vi "HEWH RLT PRAT.vi"() -> ()   [LabVIEW 2023] (continued)
        n1633 = call-poly "Enqueue Message.vi"("Priority Message? (F)"=TRUE, "error in (no error)"=w4189, "Message Data"="Temp (°F)", "Message"="Adjust_Temp_Intellifaucet_MW100", "Message Queue"=w4184) -> ("error out"=w4185:errorcluster)  [unwired: 5 in, 1 out]
      }
      frame "Adjust_Flow_Intellifaucet_MW100_UI" {
        n1634 = call-poly "Enqueue Message.vi"("Priority Message? (F)"=TRUE, "error in (no error)"=w4196, "Message Data"="Valve % Open", "Message"="Adjust_Flow_Intellifaucet_MW100", "Message Queue"=w4191) -> ("error out"=w4192:errorcluster)  [unwired: 5 in, 1 out]
      }
      frame "Adjust_Prop_Valve_MW100_UI" {
        n1635 = call-poly "Enqueue Message.vi"("Priority Message? (F)"=TRUE, "error in (no error)"=w4203, "Message Data"="Proportioning\nValve", "Message"="Adjust_Prop_Valve_MW100", "Message Queue"=w4198) -> ("error out"=w4199:errorcluster)  [unwired: 5 in, 1 out]
      }
      frame "DisplayValuesFromMW100" {
        # "Update Display - Convert the message data to a string to display in the Data Display indicator."
        n1636 = Variant To Data(error in=w4213, type=T79 {"TC1-Channel 021"=0.0, "TC2-Channel 022"=0.0, "TC3-Channel 023"=0.0, "TC4-Channel 024"=0.0, "TC5-Channel 025"=0.0, "TC6-Channel 026"=0.0, "TC7-Channel 017"=0.0, "TC8-Channel 028"=0.0, "TC9-Channel 029"=0.0, "TC10-Channel 030"=0.0, "TC Tree Average"=0.0, "TC DWN- Channel 027"=0.0, "RTDin-Channel 031"=0.0, "RTDout-Channel 032"=0.0, "RTDamb-Channel 033"=0.0, "PSI1-Channel 011"=0.0, "PSI2-Channel 012"=0.0, "PSI3-Channel 013"=0.0, "PSI4-Channel 014"=0.0, "UE State-Channel 015"=0.0, "LE State-Channel 016"=0.0, "Module 4 Relay Status Output"={"INTELLIFAUCET TEMP(T)/FLOW(F) (CH 041)"=FALSE, "INTELLIFAUCET READY (CH 042)"=FALSE, "INTELLIFAUCET START (CH 043)"=FALSE, "INTELLIFAUCET STOP (CH 044)"=FALSE, "MAIN POWER RELAY (CH 047)"=FALSE, "NOT USED (CH 045)"=FALSE, "NOT USED (CH 046)"=FALSE, "PURGE VALVE RELAY (CH 048)"=FALSE, "OUTLET VALVE RELAY (CH 049)"=FALSE, "INLET VALVE RELAY (CH 050)"=FALSE, "Intellifaucet (% Open)"=0.0, "Proportioning Valve (%Open)"=0.0, "Intellifaucet Temp Setpoint (F)"=0.0}} ("MW100 Data 2"), Variant=w4212) -> (data=w4209:T79, error out=w4207:errorcluster)
        n1637 = Bundle By Name(cluster=w4211, "MW100 Data"=w4209) -> (w4210:T67)
        n1638 = call-poly "Enqueue Message.vi"("error in (no error)"=w4207, "Message"="Process_Data", "Message Queue"=w4205) -> ("error out"=w4206:errorcluster)  [unwired: 7 in, 1 out]
        n1639 = Merge Errors(w4206) -> (w4214:errorcluster)
      }
      frame "---------- Tenney Control ----------" {
        # "Place holder, only for organization and readability"
        # "Initialize - All initialization work should take place in this message, since other loops can potentially enqueue messages that execute immediately after this one."
      }
      frame "Set_Tenney_IP_Name_UI" {
        n1640 = Variant To Data(error in=w4223, type="", Variant=w4221) -> (data=w4218:string, error out=w4222:errorcluster)
        n1641 = call-poly "Enqueue Message.vi"("Priority Message? (F)"=TRUE, "error in (no error)"=w4222, "Message Data"=w4218, "Message"="Set_Tenney_IP_Name", "Message Queue"=w4217) -> ("error out"=w4220:errorcluster)  [unwired: 5 in, 1 out]
      }
      frame "Tenney_Enable_Auto_Control_UI" {
        n1642 = Variant To Data(error in=w4231, type=TRUE, Variant=w4229) -> (data=w4228:bool, error out=w4230:errorcluster)
        n1643 = call-poly "Enqueue Message.vi"("Priority Message? (F)"=TRUE, "error in (no error)"=w4230, "Message Data"=w4228, "Message"="Tenney_Enable_Auto_Control", "Message Queue"=w4233) -> ("error out"=w4235:errorcluster)  [unwired: 5 in, 1 out]
        n1644 = Merge Errors(w4235) -> (w4236:errorcluster)
      }
      frame "PUT_Tenney_Temp_UI" {
        n1645 = call-poly "Enqueue Message.vi"("Priority Message? (F)"=TRUE, "error in (no error)"=w4243, "Message Data"="Setpoint Temperature (F)", "Message"="PUT_Tenney_Temp", "Message Queue"=w4240) -> ("error out"=w4242:errorcluster)  [unwired: 5 in, 1 out]
        n1646 = Merge Errors(w4242) -> (w4244:errorcluster)
      }
      frame "PUT_Tenney_Humidity_UI" {
        n1647 = call-poly "Enqueue Message.vi"("Priority Message? (F)"=TRUE, "error in (no error)"=w4251, "Message Data"="Setpoint Humidity (%)", "Message"="PUT_Tenney_Humidity", "Message Queue"=w4248) -> ("error out"=w4250:errorcluster)  [unwired: 5 in, 1 out]
        n1648 = Merge Errors(w4250) -> (w4252:errorcluster)
      }
      frame "PUT_Tenney_Frequency_UI" {
        n1649 = call-poly "Enqueue Message.vi"("Priority Message? (F)"=TRUE, "error in (no error)"=w4259, "Message Data"="Setpoint Frequency (Hz)", "Message"="PUT_Tenney_Frequency", "Message Queue"=w4256) -> ("error out"=w4258:errorcluster)  [unwired: 5 in, 1 out]
        n1650 = Merge Errors(w4258) -> (w4260:errorcluster)
      }
      frame "PUT_Chamber_Status_UI" {
        n1651 = Variant To Data(error in=w4266, type=Tenney_Chamber_Status."OFF" ("Chamber Status"), Variant=w4264) -> (data=w4262:T46, error out=w4265:errorcluster)
        n1652 = call-poly "Enqueue Message.vi"("Priority Message? (F)"=TRUE, "error in (no error)"=w4265, "Message Data"=w4262, "Message"="PUT_Chamber_Status", "Message Queue"=w4268) -> ("error out"=w4270:errorcluster)  [unwired: 5 in, 1 out]
        n1653 = Merge Errors(w4270) -> (w4271:errorcluster)
      }
      frame "Update_Temp_Limits_UI" {
        n1654 = call-poly "Enqueue Message.vi"("Priority Message? (F)"=TRUE, "error in (no error)"=w4274, "Message Data"="Temperature Limits", "Message"="Update_Temp_Limits", "Message Queue"=w4276) -> ("error out"=w4278:errorcluster)  [unwired: 5 in, 1 out]
        n1655 = Merge Errors(w4278) -> (w4279:errorcluster)
      }
      frame "DisplayValuesFromTenney" {
        # "Update Display - Convert the message data to a string to display in the Data Display indicator."
        n1656 = Variant To Data(error in=w4290, type=T69 {"Temperature Setpoint"=0.0, "Temperature Process Variable"=0.0, "Humidity Setpoint"=0.0, "Humidity Process Variable"=0.0, "Frequency Setpoint"=0.0, "Frequency Process Variable"=0.0, "Chamber Status (ON/OFF)"=""} ("Tenney Environmental Chamber Data"), Variant=w4289) -> (data=w4285:T69, error out=w4283:errorcluster)
        n1657 = Bundle By Name(cluster=w4287, "Tenney Data"=w4285) -> (w4286:T67)
        n1658 = call-poly "Enqueue Message.vi"("error in (no error)"=w4283, "Message"="Process_Data", "Message Queue"=w4281) -> ("error out"=w4282:errorcluster)  [unwired: 7 in, 1 out]
        n1659 = Merge Errors(w4282) -> (w4291:errorcluster)
      }
      frame "---------- GEA3 Control Station A ----------" {
        # "Place holder, only for organization and readability"
        # "Initialize - All initialization work should take place in this message, since other loops can potentially enqueue messages that execute immediately after this one."
      }
      frame "GEA3_StationA_Board_ID_UI" {
        n1660 = Variant To Data(error in=w4300, type=HEWH_GEA3_Board_ID."Board ID - 0" ("GEA3 Pink Bean Board Index (Station A)"), Variant=w4298) -> (data=w4296:T49, error out=w4299:errorcluster)
        n1661 = call-poly "Enqueue Message.vi"("Priority Message? (F)"=TRUE, "error in (no error)"=w4299, "Message Data"=w4296, "Message"="GEA3_StationA_Board_ID", "Message Queue"=w4294) -> ("error out"=w4297:errorcluster)  [unwired: 5 in, 1 out]
      }
      frame "Update_TankSP_Offset_StationA_UI" {
        n1662 = call-poly "Enqueue Message.vi"("Priority Message? (F)"=TRUE, "error in (no error)"=w4306, "Message Data"="TankSP Offset", "Message"="Update_TankSP_Offset_StationA", "Message Queue"=w4305) -> ("error out"=w4309:errorcluster)  [unwired: 5 in, 1 out]
        n1663 = Merge Errors(w4309) -> (w4310:errorcluster)
      }
      frame "Update_User_Setpoint_StationA_UI" {
        n1664 = call-poly "Enqueue Message.vi"("Priority Message? (F)"=TRUE, "error in (no error)"=w4314, "Message Data"="User Setpoint", "Message"="Update_User_Setpoint_StationA", "Message Queue"=w4313) -> ("error out"=w4317:errorcluster)  [unwired: 5 in, 1 out]
        n1665 = Merge Errors(w4317) -> (w4318:errorcluster)
      }
      frame "Update_Mode_StationA_UI" {
        n1666 = call-poly "Enqueue Message.vi"("Priority Message? (F)"=TRUE, "error in (no error)"=w4322, "Message Data"="Heating Mode.", "Message"="Update_Mode_StationA", "Message Queue"=w4321) -> ("error out"=w4325:errorcluster)  [unwired: 5 in, 1 out]
        n1667 = Merge Errors(w4325) -> (w4326:errorcluster)
      }
      frame "Update_Capacity_StationA_UI" {
        n1668 = call-poly "Enqueue Message.vi"("Priority Message? (F)"=TRUE, "error in (no error)"=w4330, "Message Data"="Capacity Setting", "Message"="Update_Capacity_StationA", "Message Queue"=w4329) -> ("error out"=w4333:errorcluster)  [unwired: 5 in, 1 out]
        n1669 = Merge Errors(w4333) -> (w4334:errorcluster)
      }
      frame "Update_Personality_StationA_UI" {
        n1670 = call-poly "Enqueue Message.vi"("Priority Message? (F)"=TRUE, "error in (no error)"=w4338, "Message Data"="Personality", "Message"="Update_Personality_StationA", "Message Queue"=w4337) -> ("error out"=w4341:errorcluster)  [unwired: 5 in, 1 out]
        n1671 = Merge Errors(w4341) -> (w4342:errorcluster)
      }
      frame "Reset_Control_Counter_StationA_UI" {
        n1672 = call-poly "Enqueue Message.vi"("Priority Message? (F)"=TRUE, "error in (no error)"=w4345, "Message"="Reset_Control_Counter_StationA", "Message Queue"=w4344) -> ("error out"=w4348:errorcluster)  [unwired: 6 in, 1 out]
        n1673 = Merge Errors(w4348) -> (w4349:errorcluster)
      }
      frame "Enable_EMV_List_StationA_UI" {
        n1674 = call-poly "Enqueue Message.vi"("Priority Message? (F)"=TRUE, "error in (no error)"=w4353, "Message Data"="Enable EMV ERD List", "Message"="Enable_EMV_List_StationA", "Message Queue"=w4352) -> ("error out"=w4356:errorcluster)  [unwired: 5 in, 1 out]
        n1675 = Merge Errors(w4356) -> (w4357:errorcluster)
      }
      frame "Enable_Inverter_List_StationA_UI" {
        n1676 = call-poly "Enqueue Message.vi"("Priority Message? (F)"=TRUE, "error in (no error)"=w4361, "Message Data"="Enable Inverter ERD List", "Message"="Enable_Inverter_List_StationA", "Message Queue"=w4360) -> ("error out"=w4364:errorcluster)  [unwired: 5 in, 1 out]
        n1677 = Merge Errors(w4364) -> (w4365:errorcluster)
      }
      frame "Enable_HeatPump_List_StationA_UI" {
        n1678 = call-poly "Enqueue Message.vi"("Priority Message? (F)"=TRUE, "error in (no error)"=w4369, "Message Data"="Enable Heat Pump ERD List", "Message"="Enable_HeatPump_List_StationA", "Message Queue"=w4368) -> ("error out"=w4372:errorcluster)  [unwired: 5 in, 1 out]
        n1679 = Merge Errors(w4372) -> (w4373:errorcluster)
      }
      frame "GEA3_Controls_UI" {
        n1680 = Variant To Data(error in=w4379, type=TRUE, Variant=w4375) -> (data=w4378:bool, error out=w4377:errorcluster)
        n1681 = case shown="True" w4378 {
          tunnel: w4377 -> [w4382 w4384]
          tunnel: [w4382 w4384] -> w4376
          frame False {
            w4383 = T87."Disabled and Grayed Out" ("Disabled")
            n1682 = property on="Update User Setpoint" class="Bool"("DisabledEnum"=w4383) -> ()  [unwired: 2 in, 2 out]
            n1683 = property on="Update Mode" class="Bool"("DisabledEnum"=w4383) -> ()  [unwired: 2 in, 2 out]
            n1684 = property on="Update TankSP Offset" class="Bool"("DisabledEnum"=w4383) -> ()  [unwired: 2 in, 2 out]
            n1685 = property on="Update Personality" class="Bool"("DisabledEnum"=w4383) -> ()  [unwired: 2 in, 2 out]
          }
          frame True {
            w4385 = T87."Enabled" ("Disabled")
            n1686 = property on="Update User Setpoint" class="Bool"("DisabledEnum"=w4385) -> ()  [unwired: 2 in, 2 out]
            n1687 = property on="Update Mode" class="Bool"("DisabledEnum"=w4385) -> ()  [unwired: 2 in, 2 out]
            n1688 = property on="Update TankSP Offset" class="Bool"("DisabledEnum"=w4385) -> ()  [unwired: 2 in, 2 out]
            n1689 = property on="Update Personality" class="Bool"("DisabledEnum"=w4385) -> ()  [unwired: 2 in, 2 out]
          }
        }
      }
      frame "DisplayValuesFromGEA_StationA" {
        # "Update Display - Convert the message data to a string to display in the Data Display indicator."
        n1690 = Variant To Data(error in=w4395, type=T76 {"ERD Data Input"={"Mixing Valve"={"T7 Temp (°F) - (0x40B9)"=0.0, "MixValveAbsoluteStepPosition - (0x400B)"=0, "Flow State - (0X4069)"=0, "T6 Temp (°F) - (0x406E)"=0.0}, "Standard ERDs"={"User UI Mode (0X4020)"="", "User Setpoint (0x4024)"=0, "Compressor (0x4068)"=FALSE, "Lower Element (0x4068)"=FALSE, "Upper Element (0x4068)"=FALSE, "Fan (0x4068)"=FALSE, "T1 Temp Lower Tank (°F) - (0x405F)"=0.0, "T2 Temp Upper Tank (°F) - (0x4060)"=0.0, "Line Voltage (0x4066)"=0, "MeasuredCurrent (0x4065)"=0.0, "Tank Setpoint (°F) - (0x4026)"=0, "Depletion - (0x40CB)"=0, "Personality - (0x0035)"=0}, "Heat Pump"={"EEV Position - (0X4067)"=0, "T3A TEMP EVAP IN (°F) - (0x4061)"=0.0, "T3B TEMP EVAP OUT (°F) -(0x4062)"=0.0, "T4 TEMP COMP DISCHARGE (°F) - (0x4063)"=0.0, "T5 TEMP AMBIENT (°F)- (0x4064)"=0.0, "Condensate Sensor - (0x40BC)"=0, "Fan (RPM) - (0xF073)"=0, "PWM (%) - (0xF056)"=0, "Compressor Speed (RPM) - (0xF093)"=0, "Compressor Target (RPM) - (0xF081)"=0, "Compressor Power (W) - (0xF092)"=0, "CPU Temperature (°F) - (0x40BA)"=0.0, "Board Temperature (°F) - (0x40BB)"=0.0}, "Inverter"={"Inverter IGBT Temp (°C) - (0xF280)"=0.0, "Inverter Chip Temp (°C) - (0xF284)"=0.0}}, "ERD Data"=[]} ("GEA3 Data"), Variant=w4394) -> (data=w4390:T76, error out=w4388:errorcluster)
        n1691 = Bundle By Name(cluster=w4392, "GEA Data - Station A"=w4390) -> (w4391:T67)
        n1692 = call-poly "Enqueue Message.vi"("error in (no error)"=w4388, "Message"="Process_Data", "Message Queue"=w4386) -> ("error out"=w4387:errorcluster)  [unwired: 7 in, 1 out]
        n1693 = Merge Errors(w4387) -> (w4396:errorcluster)
      }
      frame "---------- GEA3 Control Station B ----------" {
        # "Place holder, only for organization and readability"
        # "Initialize - All initialization work should take place in this message, since other loops can potentially enqueue messages that execute immediately after this one."
      }
      frame "GEA3_StationB_Board_ID_UI" {
        n1694 = Variant To Data(error in=w4405, type=HEWH_GEA3_Board_ID."Board ID - 0" ("GEA3 Pink Bean Board Index (Station A)"), Variant=w4403) -> (data=w4401:T49, error out=w4404:errorcluster)
        n1695 = call-poly "Enqueue Message.vi"("Priority Message? (F)"=TRUE, "error in (no error)"=w4404, "Message Data"=w4401, "Message"="GEA3_StationB_Board_ID", "Message Queue"=w4399) -> ("error out"=w4402:errorcluster)  [unwired: 5 in, 1 out]
      }
      frame "DisplayValuesFromGEA_StationB" {
        # "Update Display - Convert the message data to a string to display in the Data Display indicator."
        n1696 = Variant To Data(error in=w4418, type=T76 {"ERD Data Input"={"Mixing Valve"={"T7 Temp (°F) - (0x40B9)"=0.0, "MixValveAbsoluteStepPosition - (0x400B)"=0, "Flow State - (0X4069)"=0, "T6 Temp (°F) - (0x406E)"=0.0}, "Standard ERDs"={"User UI Mode (0X4020)"="", "User Setpoint (0x4024)"=0, "Compressor (0x4068)"=FALSE, "Lower Element (0x4068)"=FALSE, "Upper Element (0x4068)"=FALSE, "Fan (0x4068)"=FALSE, "T1 Temp Lower Tank (°F) - (0x405F)"=0.0, "T2 Temp Upper Tank (°F) - (0x4060)"=0.0, "Line Voltage (0x4066)"=0, "MeasuredCurrent (0x4065)"=0.0, "Tank Setpoint (°F) - (0x4026)"=0, "Depletion - (0x40CB)"=0, "Personality - (0x0035)"=0}, "Heat Pump"={"EEV Position - (0X4067)"=0, "T3A TEMP EVAP IN (°F) - (0x4061)"=0.0, "T3B TEMP EVAP OUT (°F) -(0x4062)"=0.0, "T4 TEMP COMP DISCHARGE (°F) - (0x4063)"=0.0, "T5 TEMP AMBIENT (°F)- (0x4064)"=0.0, "Condensate Sensor - (0x40BC)"=0, "Fan (RPM) - (0xF073)"=0, "PWM (%) - (0xF056)"=0, "Compressor Speed (RPM) - (0xF093)"=0, "Compressor Target (RPM) - (0xF081)"=0, "Compressor Power (W) - (0xF092)"=0, "CPU Temperature (°F) - (0x40BA)"=0.0, "Board Temperature (°F) - (0x40BB)"=0.0}, "Inverter"={"Inverter IGBT Temp (°C) - (0xF280)"=0.0, "Inverter Chip Temp (°C) - (0xF284)"=0.0}}, "ERD Data"=[]} ("GEA3 Data"), Variant=w4417) -> (data=w4413:T76, error out=w4411:errorcluster)
        n1697 = Bundle By Name(cluster=w4415, "GEA Data - Station B"=w4413) -> (w4414:T67)
        n1698 = call-poly "Enqueue Message.vi"("error in (no error)"=w4411, "Message"="Process_Data", "Message Queue"=w4409) -> ("error out"=w4410:errorcluster)  [unwired: 7 in, 1 out]
        n1699 = Merge Errors(w4410) -> (w4419:errorcluster)
      }
      frame "---------- GEA3 Control Station C ----------" {
        # "Place holder, only for organization and readability"
        # "Initialize - All initialization work should take place in this message, since other loops can potentially enqueue messages that execute immediately after this one."
      }
      frame "GEA3_StationC_Board_ID_UI" {
        n1700 = Variant To Data(error in=w4428, type=HEWH_GEA3_Board_ID."Board ID - 0" ("GEA3 Pink Bean Board Index (Station A)"), Variant=w4426) -> (data=w4424:T49, error out=w4427:errorcluster)
        n1701 = call-poly "Enqueue Message.vi"("Priority Message? (F)"=TRUE, "error in (no error)"=w4427, "Message Data"=w4424, "Message"="GEA3_StationC_Board_ID", "Message Queue"=w4422) -> ("error out"=w4425:errorcluster)  [unwired: 5 in, 1 out]
      }
      frame "DisplayValuesFromGEA_StationC" {
        # "Update Display - Convert the message data to a string to display in the Data Display indicator."
        n1702 = Variant To Data(error in=w4441, type=T76 {"ERD Data Input"={"Mixing Valve"={"T7 Temp (°F) - (0x40B9)"=0.0, "MixValveAbsoluteStepPosition - (0x400B)"=0, "Flow State - (0X4069)"=0, "T6 Temp (°F) - (0x406E)"=0.0}, "Standard ERDs"={"User UI Mode (0X4020)"="", "User Setpoint (0x4024)"=0, "Compressor (0x4068)"=FALSE, "Lower Element (0x4068)"=FALSE, "Upper Element (0x4068)"=FALSE, "Fan (0x4068)"=FALSE, "T1 Temp Lower Tank (°F) - (0x405F)"=0.0, "T2 Temp Upper Tank (°F) - (0x4060)"=0.0, "Line Voltage (0x4066)"=0, "MeasuredCurrent (0x4065)"=0.0, "Tank Setpoint (°F) - (0x4026)"=0, "Depletion - (0x40CB)"=0, "Personality - (0x0035)"=0}, "Heat Pump"={"EEV Position - (0X4067)"=0, "T3A TEMP EVAP IN (°F) - (0x4061)"=0.0, "T3B TEMP EVAP OUT (°F) -(0x4062)"=0.0, "T4 TEMP COMP DISCHARGE (°F) - (0x4063)"=0.0, "T5 TEMP AMBIENT (°F)- (0x4064)"=0.0, "Condensate Sensor - (0x40BC)"=0, "Fan (RPM) - (0xF073)"=0, "PWM (%) - (0xF056)"=0, "Compressor Speed (RPM) - (0xF093)"=0, "Compressor Target (RPM) - (0xF081)"=0, "Compressor Power (W) - (0xF092)"=0, "CPU Temperature (°F) - (0x40BA)"=0.0, "Board Temperature (°F) - (0x40BB)"=0.0}, "Inverter"={"Inverter IGBT Temp (°C) - (0xF280)"=0.0, "Inverter Chip Temp (°C) - (0xF284)"=0.0}}, "ERD Data"=[]} ("GEA3 Data"), Variant=w4440) -> (data=w4436:T76, error out=w4434:errorcluster)
        n1703 = Bundle By Name(cluster=w4438, "GEA Data - Station C"=w4436) -> (w4437:T67)
        n1704 = call-poly "Enqueue Message.vi"("error in (no error)"=w4434, "Message"="Process_Data", "Message Queue"=w4432) -> ("error out"=w4433:errorcluster)  [unwired: 7 in, 1 out]
        n1705 = Merge Errors(w4433) -> (w4442:errorcluster)
      }
      frame "---------- GEA3 Control Station D ----------" {
        # "Place holder, only for organization and readability"
        # "Initialize - All initialization work should take place in this message, since other loops can potentially enqueue messages that execute immediately after this one."
      }
      frame "GEA3_StationD_Board_ID_UI" {
        n1706 = Variant To Data(error in=w4451, type=HEWH_GEA3_Board_ID."Board ID - 0" ("GEA3 Pink Bean Board Index (Station A)"), Variant=w4449) -> (data=w4447:T49, error out=w4450:errorcluster)
        n1707 = call-poly "Enqueue Message.vi"("Priority Message? (F)"=TRUE, "error in (no error)"=w4450, "Message Data"=w4447, "Message"="GEA3_StationD_Board_ID", "Message Queue"=w4445) -> ("error out"=w4448:errorcluster)  [unwired: 5 in, 1 out]
      }
      frame "DisplayValuesFromGEA_StationD" {
        # "Update Display - Convert the message data to a string to display in the Data Display indicator."
        n1708 = Variant To Data(error in=w4464, type=T76 {"ERD Data Input"={"Mixing Valve"={"T7 Temp (°F) - (0x40B9)"=0.0, "MixValveAbsoluteStepPosition - (0x400B)"=0, "Flow State - (0X4069)"=0, "T6 Temp (°F) - (0x406E)"=0.0}, "Standard ERDs"={"User UI Mode (0X4020)"="", "User Setpoint (0x4024)"=0, "Compressor (0x4068)"=FALSE, "Lower Element (0x4068)"=FALSE, "Upper Element (0x4068)"=FALSE, "Fan (0x4068)"=FALSE, "T1 Temp Lower Tank (°F) - (0x405F)"=0.0, "T2 Temp Upper Tank (°F) - (0x4060)"=0.0, "Line Voltage (0x4066)"=0, "MeasuredCurrent (0x4065)"=0.0, "Tank Setpoint (°F) - (0x4026)"=0, "Depletion - (0x40CB)"=0, "Personality - (0x0035)"=0}, "Heat Pump"={"EEV Position - (0X4067)"=0, "T3A TEMP EVAP IN (°F) - (0x4061)"=0.0, "T3B TEMP EVAP OUT (°F) -(0x4062)"=0.0, "T4 TEMP COMP DISCHARGE (°F) - (0x4063)"=0.0, "T5 TEMP AMBIENT (°F)- (0x4064)"=0.0, "Condensate Sensor - (0x40BC)"=0, "Fan (RPM) - (0xF073)"=0, "PWM (%) - (0xF056)"=0, "Compressor Speed (RPM) - (0xF093)"=0, "Compressor Target (RPM) - (0xF081)"=0, "Compressor Power (W) - (0xF092)"=0, "CPU Temperature (°F) - (0x40BA)"=0.0, "Board Temperature (°F) - (0x40BB)"=0.0}, "Inverter"={"Inverter IGBT Temp (°C) - (0xF280)"=0.0, "Inverter Chip Temp (°C) - (0xF284)"=0.0}}, "ERD Data"=[]} ("GEA3 Data"), Variant=w4463) -> (data=w4459:T76, error out=w4457:errorcluster)
        n1709 = Bundle By Name(cluster=w4461, "GEA Data - Station D"=w4459) -> (w4460:T67)
        n1710 = call-poly "Enqueue Message.vi"("error in (no error)"=w4457, "Message"="Process_Data", "Message Queue"=w4455) -> ("error out"=w4456:errorcluster)  [unwired: 7 in, 1 out]
        n1711 = Merge Errors(w4456) -> (w4465:errorcluster)
      }
      frame "---------- Ultramat 23 Control ----------" {
        # "Place holder, only for organization and readability"
        # "Initialize - All initialization work should take place in this message, since other loops can potentially enqueue messages that execute immediately after this one."
      }
      frame "Set_Ultramat_VISA_Name_UI" {
        n1712 = Variant To Data(error in=w4474, type="", Variant=w4472) -> (data=w4468:string, error out=w4473:errorcluster)
        n1713 = call-poly "Enqueue Message.vi"("Priority Message? (F)"=TRUE, "error in (no error)"=w4473, "Message Data"=w4468, "Message"="Set_Ultramat_VISA_Name", "Message Queue"=w4470) -> ("error out"=w4471:errorcluster)  [unwired: 5 in, 1 out]
      }
      frame "DisplayValuesFromUltramat" {
        # "Update Display - Convert the message data to a string to display in the Data Display indicator."
        n1714 = Variant To Data(error in=w4487, type=string[][] [], Variant=w4486) -> (data=w4482:string[][], error out=w4480:errorcluster)
        n1715 = Bundle By Name(cluster=w4484, "Ultramat 23 Data"=w4482) -> (w4483:T67)
        n1716 = call-poly "Enqueue Message.vi"("error in (no error)"=w4480, "Message"="Process_Data", "Message Queue"=w4478) -> ("error out"=w4479:errorcluster)  [unwired: 7 in, 1 out]
        n1717 = Merge Errors(w4479) -> (w4488:errorcluster)
      }
      frame "---------- UI Control ----------" {
        # "Place holder, only for organization and readability"
        # "Initialize - All initialization work should take place in this message, since other loops can potentially enqueue messages that execute immediately after this one."
      }
      frame "Cancel_Draw_UI" {
        # "Initialize - All initialization work should take place in this message, since other loops can potentially enqueue messages that execute immediately after this one."
        n1718 = for {
          N: 10 -> [_]
          shift-right: [w4496] -> w4491
          shift-left: w4492 -> [w4497]
          n1719 = call "UTILITY Boolean Notifier.vi"("Status"=UTILITY_Notifier."Set", "error in (no error)"=w4497, "Set Status"=TRUE, "name (unnamed)"="Stop Custom Draw") -> ("error out"=w4496:errorcluster)  [unwired: 6 in, 1 out]
          n1720 = Wait Until Next ms Multiple(millisecond multiple=u32 10) -> ()  [unwired: 1 out]
        }
      }
      frame "DAQ_for_A_UI" {
        # "Initialize - All initialization work should take place in this message, since other loops can potentially enqueue messages that execute immediately after this one."
        n1721 = Variant To Data(error in=w4505, type=TRUE, Variant=w4501) -> (data=w4504:bool, error out=w4503:errorcluster)
        n1722 = case shown="True" w4504 {
          tunnel: w4503 -> [w4508 w4510]
          tunnel: [w4508 w4510] -> w4502
          frame False {
            w4509 = T87."Enabled" ("Disabled")
            n1723 = property on="DAQ for A" class="Bool (strict)"("DisabledEnum"=w4509) -> ()  [unwired: 2 in, 2 out]
            n1724 = property on="DAQ for B" class="Bool (strict)"("DisabledEnum"=w4509) -> ()  [unwired: 2 in, 2 out]
            n1725 = property on="DAQ for C" class="Bool (strict)"("DisabledEnum"=w4509) -> ()  [unwired: 2 in, 2 out]
            n1726 = property on="DAQ for D" class="Bool (strict)"("DisabledEnum"=w4509) -> ()  [unwired: 2 in, 2 out]
          }
          frame True {
            w4512 = T87."Disabled and Grayed Out" ("Disabled")
            n1727 = property on="DAQ for D" class="Bool (strict)"("DisabledEnum"=w4512) -> ()  [unwired: 2 in, 2 out]
            n1728 = property on="DAQ for B" class="Bool (strict)"("DisabledEnum"=w4512) -> ()  [unwired: 2 in, 2 out]
            n1729 = property on="DAQ for C" class="Bool (strict)"("DisabledEnum"=w4512) -> ()  [unwired: 2 in, 2 out]
            n1730 = property on="DAQ for A" class="Bool (strict)"("DisabledEnum"=T87."Enabled" ("Disabled")) -> ()  [unwired: 2 in, 2 out]
          }
        }
      }
      frame "DAQ_for_B_UI" {
        # "Initialize - All initialization work should take place in this message, since other loops can potentially enqueue messages that execute immediately after this one."
        n1731 = Variant To Data(error in=w4517, type=TRUE, Variant=w4513) -> (data=w4514:bool, error out=w4516:errorcluster)
        n1732 = case shown="True" w4514 {
          tunnel: w4516 -> [w4520 w4522]
          tunnel: [w4520 w4522] -> w4515
          frame False {
            w4521 = T87."Enabled" ("Disabled")
            n1733 = property on="DAQ for A" class="Bool (strict)"("DisabledEnum"=w4521) -> ()  [unwired: 2 in, 2 out]
            n1734 = property on="DAQ for B" class="Bool (strict)"("DisabledEnum"=w4521) -> ()  [unwired: 2 in, 2 out]
            n1735 = property on="DAQ for C" class="Bool (strict)"("DisabledEnum"=w4521) -> ()  [unwired: 2 in, 2 out]
            n1736 = property on="DAQ for D" class="Bool (strict)"("DisabledEnum"=w4521) -> ()  [unwired: 2 in, 2 out]
          }
          frame True {
            w4523 = T87."Disabled and Grayed Out" ("Disabled")
            n1737 = property on="DAQ for A" class="Bool (strict)"("DisabledEnum"=w4523) -> ()  [unwired: 2 in, 2 out]
            n1738 = property on="DAQ for C" class="Bool (strict)"("DisabledEnum"=w4523) -> ()  [unwired: 2 in, 2 out]
            n1739 = property on="DAQ for D" class="Bool (strict)"("DisabledEnum"=w4523) -> ()  [unwired: 2 in, 2 out]
            n1740 = property on="DAQ for B" class="Bool (strict)"("DisabledEnum"=T87."Enabled" ("Disabled")) -> ()  [unwired: 2 in, 2 out]
          }
        }
      }
      frame "DAQ_for_C_UI" {
        # "Initialize - All initialization work should take place in this message, since other loops can potentially enqueue messages that execute immediately after this one."
        n1741 = Variant To Data(error in=w4529, type=TRUE, Variant=w4525) -> (data=w4526:bool, error out=w4528:errorcluster)
        n1742 = case shown="False" w4526 {
          tunnel: w4528 -> [w4532 w4534]
          tunnel: [w4532 w4534] -> w4527
          frame False {
            w4533 = T87."Enabled" ("Disabled")
            n1743 = property on="DAQ for A" class="Bool (strict)"("DisabledEnum"=w4533) -> ()  [unwired: 2 in, 2 out]
            n1744 = property on="DAQ for D" class="Bool (strict)"("DisabledEnum"=w4533) -> ()  [unwired: 2 in, 2 out]
            n1745 = property on="DAQ for B" class="Bool (strict)"("DisabledEnum"=w4533) -> ()  [unwired: 2 in, 2 out]
            n1746 = property on="DAQ for C" class="Bool (strict)"("DisabledEnum"=w4533) -> ()  [unwired: 2 in, 2 out]
          }
          frame True {
            w4535 = T87."Disabled and Grayed Out" ("Disabled")
            n1747 = property on="DAQ for A" class="Bool (strict)"("DisabledEnum"=w4535) -> ()  [unwired: 2 in, 2 out]
            n1748 = property on="DAQ for B" class="Bool (strict)"("DisabledEnum"=w4535) -> ()  [unwired: 2 in, 2 out]
            n1749 = property on="DAQ for D" class="Bool (strict)"("DisabledEnum"=w4535) -> ()  [unwired: 2 in, 2 out]
            n1750 = property on="DAQ for C" class="Bool (strict)"("DisabledEnum"=T87."Enabled" ("Disabled")) -> ()  [unwired: 2 in, 2 out]
          }
        }
      }
      frame "DAQ_for_D_UI" {
        # "Initialize - All initialization work should take place in this message, since other loops can potentially enqueue messages that execute immediately after this one."
        n1751 = Variant To Data(error in=w4541, type=TRUE, Variant=w4537) -> (data=w4538:bool, error out=w4540:errorcluster)
        n1752 = case shown="False" w4538 {
          tunnel: w4540 -> [w4544 w4546]
          tunnel: [w4544 w4546] -> w4539
          frame False {
            w4545 = T87."Enabled" ("Disabled")
            n1753 = property on="DAQ for A" class="Bool (strict)"("DisabledEnum"=w4545) -> ()  [unwired: 2 in, 2 out]
            n1754 = property on="DAQ for B" class="Bool (strict)"("DisabledEnum"=w4545) -> ()  [unwired: 2 in, 2 out]
            n1755 = property on="DAQ for C" class="Bool (strict)"("DisabledEnum"=w4545) -> ()  [unwired: 2 in, 2 out]
            n1756 = property on="DAQ for D" class="Bool (strict)"("DisabledEnum"=w4545) -> ()  [unwired: 2 in, 2 out]
          }
          frame True {
            w4548 = T87."Disabled and Grayed Out" ("Disabled")
            n1757 = property on="DAQ for A" class="Bool (strict)"("DisabledEnum"=w4548) -> ()  [unwired: 2 in, 2 out]
            n1758 = property on="DAQ for B" class="Bool (strict)"("DisabledEnum"=w4548) -> ()  [unwired: 2 in, 2 out]
            n1759 = property on="DAQ for C" class="Bool (strict)"("DisabledEnum"=w4548) -> ()  [unwired: 2 in, 2 out]
            n1760 = property on="DAQ for D" class="Bool (strict)"("DisabledEnum"=T87."Enabled" ("Disabled")) -> ()  [unwired: 2 in, 2 out]
          }
        }
      }
      frame "Change_Gas_UI" {
        n1761 = call-poly "Enqueue Message.vi"("Priority Message? (F)"=TRUE, "error in (no error)"=w4559, "Message Data"="Gas Type", "Message"="Alicat_Change_Gas", "Message Queue"=w4555) -> ("error out"=w4553:errorcluster)  [unwired: 5 in, 1 out]
        n1762 = call-poly "Enqueue Message.vi"("Priority Message? (F)"=TRUE, "error in (no error)"=w4553, "Message Data"="Gas Type", "Message"="Ultramat_Select_Gas", "Message Queue"=w4551) -> ("error out"=w4552:errorcluster)  [unwired: 5 in, 1 out]
      }
      frame "Update_Graph_StationA_UI" {
        (unwired) 0 ("disabled index (col)")
        (unwired) 0 ("disabled index (col)")
        (unwired) 0 ("disabled index (col)")
        # "Initialize - All initialization work should take place in this message, since other loops can potentially enqueue messages that execute immediately after this one."
        n1763 = local read "Station A"() -> (w4562:string[][])
        n1764 = Transpose 2D Array(2D array=w4562) -> (transposed array=w4561:string[][])
        n1765 = Index Array(array=w4561) -> (element=w4565:string[])  [unwired: 2 in]
        n1766 = Index Array(array=w4561) -> (element=w4564:string[])  [unwired: 2 in]
        n1767 = Index Array(array=w4561) -> (element=w4563:string[])  [unwired: 2 in]
        n1768 = property on="X-Axis - Station A" class="CmbBox"("Strings[]"=w4565) -> ()  [unwired: 2 in, 2 out]
        n1769 = property on="Y-Axis1 - Station A" class="CmbBox"("Strings[]"=w4564) -> ()  [unwired: 2 in, 2 out]
        n1770 = property on="Y-Axis2 - Station A" class="CmbBox"("Strings[]"=w4563) -> ()  [unwired: 2 in, 2 out]
      }
      frame "Update_Graph_StationB_UI" {
        (unwired) 0 ("disabled index (col)")
        (unwired) 0 ("disabled index (col)")
        (unwired) 0 ("disabled index (col)")
        # "Initialize - All initialization work should take place in this message, since other loops can potentially enqueue messages that execute immediately after this one."
        n1771 = local read "Station B"() -> (w4568:string[][])
        n1772 = Transpose 2D Array(2D array=w4568) -> (transposed array=w4567:string[][])
        n1773 = Index Array(array=w4567) -> (element=w4571:string[])  [unwired: 2 in]
        n1774 = Index Array(array=w4567) -> (element=w4570:string[])  [unwired: 2 in]
        n1775 = Index Array(array=w4567) -> (element=w4569:string[])  [unwired: 2 in]
        n1776 = property on="X-Axis - Station B" class="CmbBox"("Strings[]"=w4571) -> ()  [unwired: 2 in, 2 out]
        n1777 = property on="Y-Axis1 - Station B" class="CmbBox"("Strings[]"=w4570) -> ()  [unwired: 2 in, 2 out]
        n1778 = property on="Y-Axis2 - Station B" class="CmbBox"("Strings[]"=w4569) -> ()  [unwired: 2 in, 2 out]
      }
      frame "Update_Graph_StationC_UI" {
        (unwired) 0 ("disabled index (col)")
        (unwired) 0 ("disabled index (col)")
        (unwired) 0 ("disabled index (col)")
        # "Initialize - All initialization work should take place in this message, since other loops can potentially enqueue messages that execute immediately after this one."
        n1779 = local read "Station C"() -> (w4575:string[][])
        n1780 = Transpose 2D Array(2D array=w4575) -> (transposed array=w4574:string[][])
        n1781 = Index Array(array=w4574) -> (element=w4578:string[])  [unwired: 2 in]
        n1782 = Index Array(array=w4574) -> (element=w4577:string[])  [unwired: 2 in]
        n1783 = Index Array(array=w4574) -> (element=w4576:string[])  [unwired: 2 in]
        n1784 = property on="X-Axis - Station C" class="CmbBox"("Strings[]"=w4578) -> ()  [unwired: 2 in, 2 out]
        n1785 = property on="Y-Axis1 - Station C" class="CmbBox"("Strings[]"=w4577) -> ()  [unwired: 2 in, 2 out]
        n1786 = property on="Y-Axis2 - Station C" class="CmbBox"("Strings[]"=w4576) -> ()  [unwired: 2 in, 2 out]
      }
      frame "Update_Graph_StationD_UI" {
        (unwired) 0 ("disabled index (col)")
        (unwired) 0 ("disabled index (col)")
        (unwired) 0 ("disabled index (col)")
        # "Initialize - All initialization work should take place in this message, since other loops can potentially enqueue messages that execute immediately after this one."
        n1787 = local read "Station D"() -> (w4581:string[][])
        n1788 = Transpose 2D Array(2D array=w4581) -> (transposed array=w4582:string[][])
        n1789 = Index Array(array=w4582) -> (element=w4585:string[])  [unwired: 2 in]
        n1790 = Index Array(array=w4582) -> (element=w4584:string[])  [unwired: 2 in]
        n1791 = Index Array(array=w4582) -> (element=w4583:string[])  [unwired: 2 in]
        n1792 = property on="X-Axis - Station D" class="CmbBox"("Strings[]"=w4585) -> ()  [unwired: 2 in, 2 out]
        n1793 = property on="Y-Axis1 - Station D" class="CmbBox"("Strings[]"=w4584) -> ()  [unwired: 2 in, 2 out]
        n1794 = property on="Y-Axis2 - Station D" class="CmbBox"("Strings[]"=w4583) -> ()  [unwired: 2 in, 2 out]
      }
      frame "---------- Alicat Gas Meter ----------" {
        # "Place holder, only for organization and readability"
        # "Initialize - All initialization work should take place in this message, since other loops can potentially enqueue messages that execute immediately after this one."
      }
      frame "Set_Alicat_VISA_Name_UI" {
        n1795 = Variant To Data(error in=w4596, type="", Variant=w4594) -> (data=w4591:string, error out=w4595:errorcluster)
        n1796 = call-poly "Enqueue Message.vi"("Priority Message? (F)"=TRUE, "error in (no error)"=w4595, "Message Data"=w4591, "Message"="Set_Alicat_VISA_Name", "Message Queue"=w4590) -> ("error out"=w4593:errorcluster)  [unwired: 5 in, 1 out]
      }
      frame "Alicat_Tare_Flow_UI" {
        n1797 = call-poly "Enqueue Message.vi"("Priority Message? (F)"=TRUE, "error in (no error)"=w4605, "Message"="Alicat_Tare_Flow", "Message Queue"=w4601) -> ("error out"=w4600:errorcluster)  [unwired: 6 in, 1 out]
      }
      frame "DisplayValuesFromAlicat" {
        # "Update Display - Convert the message data to a string to display in the Data Display indicator."
        n1798 = Variant To Data(error in=w4615, type=T71 {"Data Cluster"={"Absolute Pressure"=0.0, "Gauge/Diff. Pressure"=0.0, "Barometric Pressure"=0.0, "Temperature"=0.0, "Volumetric Flow"=0.0, "Mass Flow"=0.0, "Setpoint"=0.0, "Valve Drive"=0.0, "Totalizer"=0.0, "[hr]"=0.0, "[min]"=0.0, "[sec]"=0.0, "Totalizer Average Flow"=0.0, "Totalizer Peak Flow"=0.0, "Gas selected"=""}, "Units of Measure Input"={"Abs. Pressure"="", "Gauge/Diff. Press."="", "Barometric Press."="", "Temperature"="", "Volume"="", "Mass"="", "Setpoint"="", "Valve Drive"="", "Totalizer"="", "Tot. Timer"="", "Tot. Avg. Flow"="", "Tot. Peak Flow"=""}, "Header Array"=[]} ("Gas Data"), Variant=w4614) -> (data=w4610:T71, error out=w4608:errorcluster)
        n1799 = Bundle By Name(cluster=w4612, "Alicat Data"=w4610) -> (w4611:T67)
        n1800 = call-poly "Enqueue Message.vi"("error in (no error)"=w4608, "Message"="Process_Data", "Message Queue"=w4606) -> ("error out"=w4607:errorcluster)  [unwired: 7 in, 1 out]
        n1801 = Merge Errors(w4607) -> (w4616:errorcluster)
      }
      frame "---------- Wet Gas Meter ----------" {
        # "Place holder, only for organization and readability"
        # "Initialize - All initialization work should take place in this message, since other loops can potentially enqueue messages that execute immediately after this one."
      }
      frame "Set_Ritter_VISA_Name_UI" {
        n1802 = Variant To Data(error in=w4625, type="", Variant=w4623) -> (data=w4620:string, error out=w4624:errorcluster)
        n1803 = call-poly "Enqueue Message.vi"("Priority Message? (F)"=TRUE, "error in (no error)"=w4624, "Message Data"=w4620, "Message"="Set_Ritter_VISA_Name", "Message Queue"=w4619) -> ("error out"=w4622:errorcluster)  [unwired: 5 in, 1 out]
      }
      frame "Reset_Gas_Totalizer_UI" {
        w4633 = TRUE ("Priority Message? (F)")
        n1804 = call-poly "Enqueue Message.vi"("Priority Message? (F)"=w4633, "error in (no error)"=w4637, "Message"="Alicat_Tare_Totalizer", "Message Queue"=w4630) -> ("error out"=w4635:errorcluster)  [unwired: 6 in, 1 out]
        n1805 = call-poly "Enqueue Message.vi"("Priority Message? (F)"=w4633, "error in (no error)"=w4635, "Message"="Ritter_Tare_Totalizer", "Message Queue"=w4629) -> ("error out"=w4634:errorcluster)  [unwired: 6 in, 1 out]
      }
      frame "DisplayValuesFromRitter" {
        w4645 = T1 {"Gas Flow Rate (L/hr)-Uncorrected"=0.0, "Totalized Flow (L)--Uncorrected"=0.0, "Gas Flow Rate (cuft/hr)-Uncorrected"=0.0, "Totalized Flow (cuft)-Uncorrected"=0.0, "Gas Temperature (F)"=0.0, "Gas Pressure (in WC)"=0.0, "Heise Barometric Pressure (inHG)"=0.0, "STP Correction Factor"=0.0, "Temp Correction Factor"=0.0, "Pressure Correction Factor"=0.0, "Water Vapor Pressure"=0.0, "Gas Flow Rate (cuft/hr)-Corrected"=0.0, "Totalized Flow (cuft)-Corrected"=0.0, "Gas BTU"=0.0, "Gas BTU/hr"=0.0, "Gas Flow Rate (cuft/hr)-Uncorrected-Raw"=0.0}  # Gas Measurment Data - Ritter
        # "Update Display - Convert the message data to a string to display in the Data Display indicator."
        n1806 = Variant To Data(error in=w4647, type=w4645, Variant=w4646) -> (data=w4642:T1, error out=w4640:errorcluster)
        n1807 = Bundle By Name(cluster=w4644, "Ritter Data"=w4642) -> (w4643:T67)
        n1808 = call-poly "Enqueue Message.vi"("error in (no error)"=w4640, "Message"="Process_Data", "Message Queue"=w4638) -> ("error out"=w4639:errorcluster)  [unwired: 7 in, 1 out]
        n1809 = Merge Errors(w4639) -> (w4648:errorcluster)
      }
      frame "---------- Laurel Water Meter Control ----------" {
        # "Place holder, only for organization and readability"
        # "Initialize - All initialization work should take place in this message, since other loops can potentially enqueue messages that execute immediately after this one."
      }
      frame "Set_Laurel_IP_Name_UI" {
        n1810 = Variant To Data(error in=w4657, type="", Variant=w4655) -> (data=w4652:string, error out=w4656:errorcluster)
        n1811 = call-poly "Enqueue Message.vi"("Priority Message? (F)"=TRUE, "error in (no error)"=w4656, "Message Data"=w4652, "Message"="Set_Laurel_IP_Name", "Message Queue"=w4651) -> ("error out"=w4654:errorcluster)  [unwired: 5 in, 1 out]
      }
      frame "DisplayValuesFromLaurel" {
        # "Update Display - Convert the message data to a string to display in the Data Display indicator."
        n1812 = Variant To Data(error in=w4670, type=T73 {"Flow Rate (GPM)"=0.0, "Totalized Flow (Gallons)"=0.0} ("Laurel Meter Data"), Variant=w4669) -> (data=w4665:T73, error out=w4663:errorcluster)
        n1813 = Bundle By Name(cluster=w4667, "Laurel Meter Data"=w4665) -> (w4666:T67)
        n1814 = call-poly "Enqueue Message.vi"("error in (no error)"=w4663, "Message"="Process_Data", "Message Queue"=w4661) -> ("error out"=w4662:errorcluster)  [unwired: 7 in, 1 out]
        n1815 = Merge Errors(w4662) -> (w4671:errorcluster)
      }
      frame "---------- Emerson Water Meter Control ----------" {
        # "Place holder, only for organization and readability"
        # "Initialize - All initialization work should take place in this message, since other loops can potentially enqueue messages that execute immediately after this one."
      }
      frame "Set_Emerson_IP_Name_UI" {
        n1816 = Variant To Data(error in=w4680, type="", Variant=w4678) -> (data=w4675:string, error out=w4679:errorcluster)
        n1817 = call-poly "Enqueue Message.vi"("Priority Message? (F)"=TRUE, "error in (no error)"=w4679, "Message Data"=w4675, "Message"="Set_Emerson_IP_Name", "Message Queue"=w4674) -> ("error out"=w4677:errorcluster)  [unwired: 5 in, 1 out]
      }
      frame "Reset_Inventory_Emerson_UI" {
        n1818 = call-poly "Enqueue Message.vi"("Priority Message? (F)"=TRUE, "error in (no error)"=w4689, "Message"="Reset_Inventory_Emerson", "Message Queue"=w4684) -> ("error out"=w4685:errorcluster)  [unwired: 6 in, 1 out]
      }
      frame "Reset_Totalizer_UI" {
        n1819 = call-poly "Enqueue Message.vi"("Priority Message? (F)"=TRUE, "error in (no error)"=w4699, "Message"="Reset_Totalizer_Emerson", "Message Queue"=w4695) -> ("error out"=w4692:errorcluster)  [unwired: 6 in, 1 out]
        n1820 = call-poly "Enqueue Message.vi"("Priority Message? (F)"=TRUE, "error in (no error)"=w4692, "Message"="Reset_Totalizer_Laurel", "Message Queue"=w4690) -> ("error out"=w4691:errorcluster)  [unwired: 6 in, 1 out]
      }
      frame "DisplayValuesFromEmerson" {
        # "Update Display - Convert the message data to a string to display in the Data Display indicator."
        n1821 = Variant To Data(error in=w4709, type=T72 {"Mass Flow Rate (Scaled Integer)"=0, "Density (Scaled Integer)"=0, "Temperature (Scaled Integer)"=0, "Volume Flow Rate (Scaled Integer)"=0, "Totalizer 1 (Scaled Integer)"=0, "Totalizer 2 (Scaled Integer)"=0, "Transmitter Software Rev"=0, "Flow Direction"="", "Mass Flow Units"="", "Density Units"="", "Temperature Units"="", "Volume Flow Units"="", "Pressure Units"="", "Mass Total Units"="", "Volume Total Units"="", "Inventory 1 (Scaled Integer)"=0, "Inventory 2 (Scaled Integer)"=0, "Mass Flow Rate"=0.0, "Density"=0.0, "Temperature"=0.0, "Volume Flow Rate"=0.0, "Pressure (Scaled Integer)"=0, "Current Value Totalizer 1 (Pounds per draw)"=0.0, "Current Value Totalizer 2 (Gallons per draw)"=0.0, "Current Value Inventory 1 (Pounds Total)"=0.0, "Current Value Inventory 2 (Gallons Total)"=0.0, "Drive Gain"=0.0, "Raw Tube Frequency (Hz)"=0.0, "Dynamic Viscosity (Centipoise)"=0.0, "Kinematic Viscosity (Centistokes)"=0.0, "Hot Gallons (Calculated Gallons)"=0.0, "Hot Flow Rate (Calculated GPM)"=0.0, "Hot Gallons Inventory (Gallons)"=0.0, "Hot Flow Rate (Laurel)"=0.0, "Hot Gallons (Laurel)"=0.0} ("Emerson Flow Meter Data Output"), Variant=w4708) -> (data=w4704:T72, error out=w4702:errorcluster)
        n1822 = Bundle By Name(cluster=w4706, "Emerson Data"=w4704) -> (w4705:T67)
        n1823 = call-poly "Enqueue Message.vi"("error in (no error)"=w4702, "Message"="Process_Data", "Message Queue"=w4700) -> ("error out"=w4701:errorcluster)  [unwired: 7 in, 1 out]
        n1824 = Merge Errors(w4701) -> (w4710:errorcluster)
      }
      frame "---------- Power Analyzer Control ----------" {
        # "Place holder, only for organization and readability"
        # "Initialize - All initialization work should take place in this message, since other loops can potentially enqueue messages that execute immediately after this one."
      }
      frame "Set_WT300_VISA_Name_UI" {
        n1825 = Variant To Data(error in=w4719, type="", Variant=w4717) -> (data=w4714:string, error out=w4718:errorcluster)
        n1826 = call-poly "Enqueue Message.vi"("Priority Message? (F)"=TRUE, "error in (no error)"=w4718, "Message Data"=w4714, "Message"="Set_WT300_VISA_Name", "Message Queue"=w4713) -> ("error out"=w4716:errorcluster)  [unwired: 5 in, 1 out]
      }
      frame "Reset_PowerAnalyzer_UI" {
        # "Do i need to reset MW100 here also? \nDo think so...but verify"
        n1827 = call-poly "Enqueue Message.vi"("Priority Message? (F)"=TRUE, "error in (no error)"=w4724, "Message"="Reset_WT300", "Message Queue"=w4723) -> ("error out"=w4725:errorcluster)  [unwired: 6 in, 1 out]
      }
      frame "DisplayValuesFromWT300" {
        # "Update Display - Convert the message data to a string to display in the Data Display indicator."
        n1828 = Variant To Data(error in=w4738, type=T74 {"Current (A):Element 1"=236.2, "Current (A):Element 2"=17.749, "Power (W):Sigma"=4192.0, "Watt Hours (Wh):Sigma"=0.0, "Voltage (V):Element 2"=236.2, "Voltage (V):Element 1"=236.2, "Current Crest Factor:Element 1"=0.0, "Current Crest Factor:Element 2"=0.0, "Voltage Harmonic (%):Element 1"=0.0, "Voltage Harmonic (%):Element 2"=0.0, "Voltage Crest Factor:Element 1"=0.0, "Voltage Crest Factor:Element 2"=0.0, "Time:Element 1"=0.0, "Frequency (Hz):Element 1"=0.0, "Apparent Power (VA):Element 1"=0.0, "Apparent Power (VA):Element 2"=0.0, "Power Factor:Element 1"=0.0, "Power Factor:Element 2"=0.0, "Max Watt Hours"=0.0, "Voltage (V):Element 2 Avg"=0.0, "Voltage (V):Element 1 Avg"=0.0} ("Power Data"), Variant=w4737) -> (data=w4733:T74, error out=w4731:errorcluster)
        n1829 = Bundle By Name(cluster=w4735, "WT300 Data"=w4733) -> (w4734:T67)
        n1830 = call-poly "Enqueue Message.vi"("error in (no error)"=w4731, "Message"="Process_Data", "Message Queue"=w4729) -> ("error out"=w4730:errorcluster)  [unwired: 7 in, 1 out]
        n1831 = Merge Errors(w4730) -> (w4739:errorcluster)
      }
      frame "---------- NG Inficon Control ----------" {
        # "Place holder, only for organization and readability"
        # "Initialize - All initialization work should take place in this message, since other loops can potentially enqueue messages that execute immediately after this one."
      }
      frame "Set_NG_Inficon_IP_Name_UI" {
        n1832 = Variant To Data(error in=w4748, type="", Variant=w4746) -> (data=w4743:string, error out=w4747:errorcluster)
        n1833 = call-poly "Enqueue Message.vi"("Priority Message? (F)"=TRUE, "error in (no error)"=w4747, "Message Data"=w4743, "Message"="Set_NG_Inficon_IP_Name", "Message Queue"=w4742) -> ("error out"=w4745:errorcluster)  [unwired: 5 in, 1 out]
      }
      frame "Manual_Heating_Value_UI" {
        # "Need to add the HHV value setting"
        n1834 = Variant To Data(error in=w4757, type=TRUE, Variant=w4755) -> (data=w4754:bool, error out=w4756:errorcluster)
        n1835 = call "Inficon_Manual_HHV.vi"("HHV-NG-Manual"="HHV-NG-Manual", "Manual HHV"=w4754, "HHV-LP-Manual"="HHV-LP-Manual", "error in (no error)"=w4756, "Inficon_LP"=w4759, "Inficon_NG"=w4761) -> ("error out"=w4760:errorcluster)  [unwired: 5 in]
      }
      frame "Heating_Value_Adjust_NG_UI" {
        n1836 = Variant To Data(error in=w4769, type=0.0, Variant=w4767) -> (data=w4766:dbl, error out=w4768:errorcluster)
        n1837 = call-poly "Enqueue Message.vi"("Priority Message? (F)"=TRUE, "error in (no error)"=w4768, "Message Data"=w4766, "Message"="Heating_Value_Adjust_NG", "Message Queue"=w4763) -> ("error out"=w4765:errorcluster)  [unwired: 5 in, 1 out]
      }
      frame "DisplayValuesFromInficon" {
        # "Update Display - Convert the message data to a string to display in the Data Display indicator."
        n1838 = Variant To Data(error in=w4782, type=T53 {"Gross Heating Value, Vol (Real, Dry)"=0.0, "Nitrogen Component Normalized Mole % (Dry)"=0.0, "Methane Component Normalized Mole % (Dry)"=0.0, "Carbon Dioxide Component Normalized Mole % (Dry)"=0.0, "Ethane Component Normalized Mole % (Dry)"=0.0, "Propane Component Normalized Mole % (Dry)"=0.0, "i-Pentane Component Normalized Mole % (Dry)"=0.0, "i-Butane Component Normalized Mole % (Dry)"=0.0, "n-Butane Component Normalized Mole % (Dry)"=0.0, "n-Pentane Component Normalized Mole % (Dry)"=0.0, "Hexane Component Normalized Mole % (Dry)"=0.0, "Heptane Component Normalized Mole % (Dry)"=0.0, "Gross Wobbe Index, Real(Dry)"=0.0, "Relative Density, Real(Dry)"=0.0, "Propylene Component Normalized Mole % (Dry)"=0.0, "C4 Olefins Component Normalized Mole % (Dry)"=0.0, "Water Component Normalized Mole % (Dry)"=0.0, "Gross Heating Value, Vol (Real, Sat)"=0.0, "Natural Gas Data"=[], "Propane Data"=[]} ("Inficon Data Input"), Variant=w4781) -> (data=w4777:T53, error out=w4775:errorcluster)
        n1839 = Bundle By Name(cluster=w4779, "Inficon Data"=w4777) -> (w4778:T67)
        n1840 = call-poly "Enqueue Message.vi"("error in (no error)"=w4775, "Message"="Process_Data", "Message Queue"=w4773) -> ("error out"=w4774:errorcluster)  [unwired: 7 in, 1 out]
        n1841 = Merge Errors(w4774) -> (w4783:errorcluster)
      }
      frame "---------- LP Inficon Control ----------" {
        # "Place holder, only for organization and readability"
        # "Initialize - All initialization work should take place in this message, since other loops can potentially enqueue messages that execute immediately after this one."
      }
      frame "Set_LP_Inficon_IP_Name_UI" {
        n1842 = Variant To Data(error in=w4792, type="", Variant=w4790) -> (data=w4787:string, error out=w4791:errorcluster)
        n1843 = call-poly "Enqueue Message.vi"("Priority Message? (F)"=TRUE, "error in (no error)"=w4791, "Message Data"=w4787, "Message"="Set_LP_Inficon_IP_Name", "Message Queue"=w4786) -> ("error out"=w4789:errorcluster)  [unwired: 5 in, 1 out]
      }
